vi "Get Time Ref Properties.vi"(8 "error in (no error)":errorcluster, 10 "TimeKeeper Module":string, 11 "Device Item Ref in":T1 format="%.0x") -> (0 "error out":errorcluster, 2 "Time Ref Settings":T2={"Time Reference"=enum."GPS", "Priority 1"=0, "Priority 2"=0, "IRIG type"=enum."IRIGB AM", "Terminal"="", "PPSSetTime"=FALSE, "Start Time"=timestamp(0 s since 1904-01-01)} {"Priority 2" min=0 max=255; "Priority 1" min=0 max=255}, 3 "Item Ref out":T1 format="%.0x")   [LabVIEW 2015, in "NI Synchronization System Explorer.lvlib"]
uses:
  NI Synchronization System Explorer.lvlib
  Shared/Time Ref Settings.ctl
  Shared/Time Reference.ctl
  Shared/IRIG Type.ctl
  <vilib>/NI Veristand/Custom Device API/Custom Device Item Ref.ctl
  Shared/Constants.vi
  <vilib>/NI Veristand/Custom Device API/Get Item Property (U16).vi
  <vilib>/NI Veristand/Custom Device API/Get Item Property (I32).vi
  <vilib>/NI Veristand/Custom Device API/Get Item Property (String).vi
  <vilib>/NI Veristand/Custom Device API/Get Item Property (Boolean).vi
  <vilib>/NI Veristand/Custom Device API/Get Item Property (Variant).vi
  <vilib>/NI Veristand/Custom Device API/Custom Device API.lvlib
  Shared/NI Synchronization Shared.lvlib
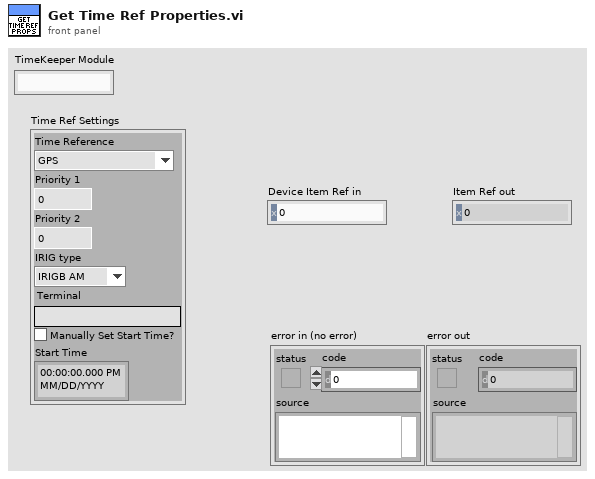
[diagram p1: front panel]
types:
  T1 = typedef "Custom Device API.lvlib/Custom Device Item Ref.ctl" = u64
  T2 = typedef "NI Synchronization Shared.lvlib/Time Ref Settings.ctl" = cluster{"Time Reference":T3, "Priority 1":i32, "Priority 2":i32, "IRIG type":T4, "Terminal":string, "PPSSetTime":bool, "Start Time":timestamp}
  T3 = typedef "NI Synchronization Shared.lvlib/Time Reference.ctl" = enum16{"GPS", "IRIG", "PPS", "1588 Ordinary Clock", "802.1AS", "PXI Chassis Clock", "Free Running (Internal)"}
  T4 = typedef "NI Synchronization Shared.lvlib/IRIG Type.ctl" = enum16{"IRIGB DC", "IRIGB AM"}
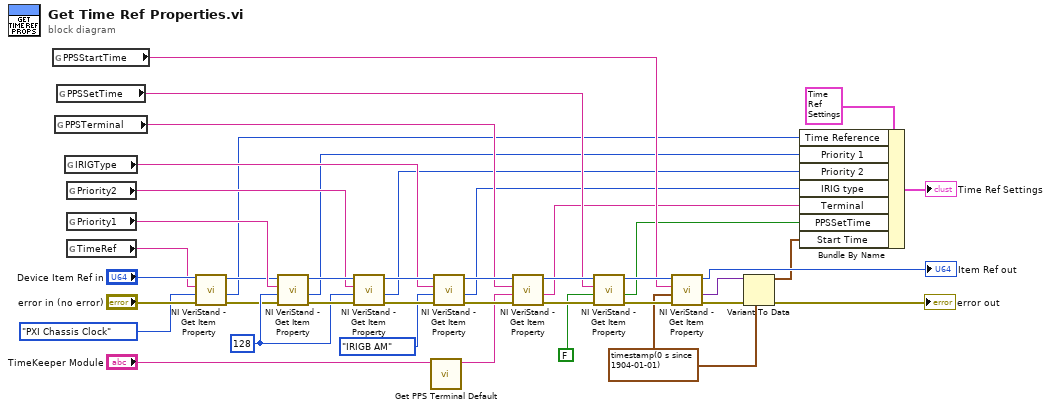
[diagram p0: block diagram]
diagram:
  w9 = 128 ("Priority 2")
  w18 = timestamp(0 s since 1904-01-01) ("Start Time")
  n1 = global read "Constants.vi" "PPSStartTime"() -> (w23:string)
  n2 = global read "Constants.vi" "PPSTerminal"() -> (w29:string)
  n3 = global read "Constants.vi" "PPSSetTime"() -> (w26:string)
  n4 = global read "Constants.vi" "IRIGType"() -> (w32:string)
  n5 = global read "Constants.vi" "Priority2"() -> (w35:string)
  n6 = global read "Constants.vi" "Priority1"() -> (w38:string)
  n7 = global read "Constants.vi" "TimeRef"() -> (w4:string)
  n8 = call-poly <vilib>:"NI VeriStand - Get Item Property.vi"("error in (no error)"="error in (no error)", "Default Value"=Time_Reference."PXI Chassis Clock" ("Time Reference"), "Property Name"=w4, "Item Ref in"="Device Item Ref in") -> ("error out"=w7:errorcluster, "Value"=w3:u16, "Item Ref out"=w5:T1)  [unwired: 4 in, 1 out]
  n9 = call-poly <vilib>:"NI VeriStand - Get Item Property.vi"("error in (no error)"=w7, "Default Value"=w9, "Property Name"=w38, "Item Ref in"=w5) -> ("error out"=w36:errorcluster, "Value"=w8:i32, "Item Ref out"=w37:T1)  [unwired: 4 in, 1 out]
  n10 = call-poly <vilib>:"NI VeriStand - Get Item Property.vi"("error in (no error)"=w36, "Default Value"=w9, "Property Name"=w35, "Item Ref in"=w37) -> ("error out"=w33:errorcluster, "Value"=w10:i32, "Item Ref out"=w34:T1)  [unwired: 4 in, 1 out]
  n11 = call "Get PPS Terminal Default.vi"("TimeKeeper Module"="TimeKeeper Module") -> ("PPSTerminal Default"=w14:string)  [unwired: 10 in]
  n12 = call-poly <vilib>:"NI VeriStand - Get Item Property.vi"("error in (no error)"=w33, "Default Value"=IRIG_Type."IRIGB AM" ("IRIG type"), "Property Name"=w32, "Item Ref in"=w34) -> ("error out"=w30:errorcluster, "Value"=w11:u16, "Item Ref out"=w31:T1)  [unwired: 4 in, 1 out]
  n13 = call-poly <vilib>:"NI VeriStand - Get Item Property.vi"("error in (no error)"=w30, "Default Value"=w14, "Property Name"=w29, "Item Ref in"=w31) -> ("error out"=w27:errorcluster, "Value"=w13:string, "Item Ref out"=w28:T1)  [unwired: 4 in, 1 out]
  n14 = call-poly <vilib>:"NI VeriStand - Get Item Property.vi"("error in (no error)"=w27, "Default Value"=FALSE, "Property Name"=w26, "Item Ref in"=w28) -> ("error out"=w25:errorcluster, "Value"=w16:bool, "Item Ref out"=w24:T1)  [unwired: 4 in, 1 out]
  n15 = call-poly <vilib>:"NI VeriStand - Get Item Property.vi"("error in (no error)"=w25, "Default Value"=w18, "Property Name"=w23, "Item Ref in"=w24) -> ("error out"=w22:errorcluster, "Value"=w19:variant, "Item Ref out"=→"Item Ref out":T1)  [unwired: 4 in, 1 out]
  n16 = Variant To Data(error in=w22, type=w18, Variant=w19) -> (data=w17:timestamp, error out=→"error out":errorcluster)
  n17 = Bundle By Name(cluster=T2 {"Time Reference"=enum."GPS", "Priority 1"=0, "Priority 2"=0, "IRIG type"=enum."IRIGB AM", "Terminal"="", "PPSSetTime"=FALSE, "Start Time"=timestamp(0 s since 1904-01-01)}, "Time Reference"=w3, "Priority 1"=w8, "Priority 2"=w10, "IRIG type"=w11, "Terminal"=w13, "PPSSetTime"=w16, "Start Time"=w17) -> (→"Time Ref Settings":T2)
